vi "WM Dispersion Solver.vi"(1 "Gravity":dbl=9.806 min=1.0 format="%.3f", 2 "Water Depth":dbl=2.438 min=1e-16 format="%.3f", 3 "Wave Period":dbl=1.0 min=1e-16 format="%.3f") -> (0 "Wave Length":dbl format="%.3e")   [LabVIEW 2012]
uses:
  <vilib>/gmath/NI_Gmath.lvlib
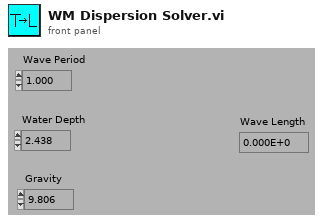
[diagram p1: front panel]
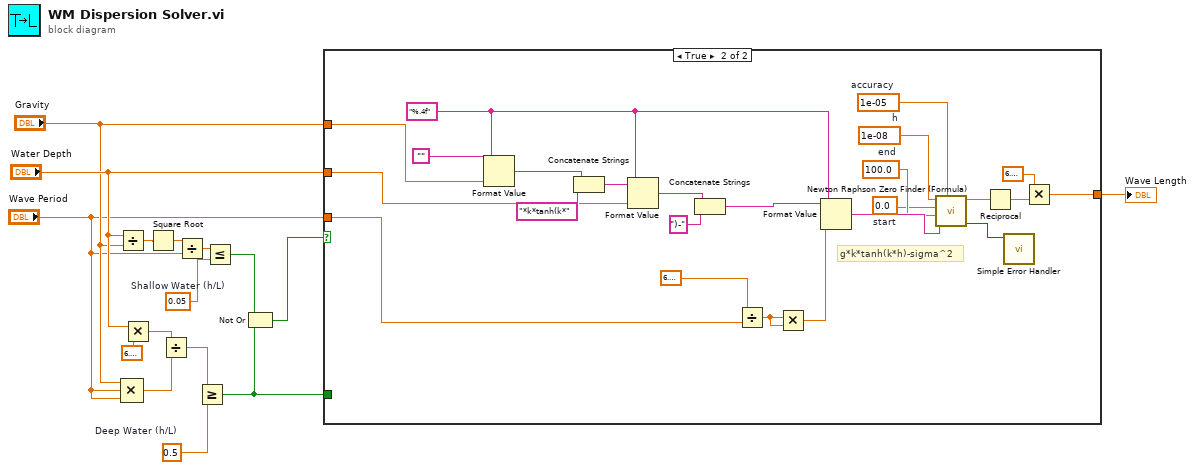
[diagram p0: block diagram]
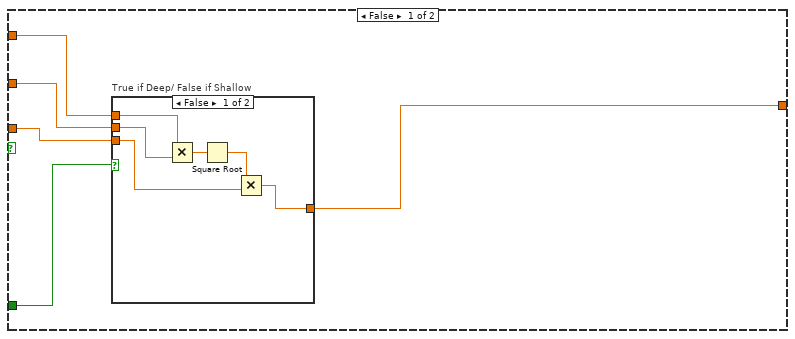
[diagram p2: hidden frame]
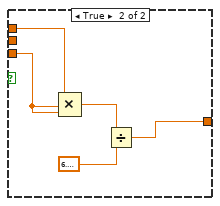
[diagram p3: hidden frame]
diagram:
  w5 = 0.5  # Deep Water (h/L)
  w12 = 0.05  # Shallow Water (h/L)
  n1 = Divide(x="Water Depth", y="Gravity") -> (x/y=w15:dbl)
  n2 = Compound Arithmetic op=MULTIPLY("Gravity", "Wave Period", "Wave Period") -> (w6:dbl)
  n3 = Multiply(x="Water Depth", y=6.283185307179586) -> (x*y=w9:dbl)
  n4 = Square Root(x=w15) -> (sqrt(x)=w14:dbl)
  n5 = Divide(x=w9, y=w6) -> (x/y=w4:dbl)
  n6 = Divide(x=w14, y="Wave Period") -> (x/y=w13:dbl)
  n7 = Greater Or Equal?(x=w4, y=w5) -> (x >= y?=w1:bool)
  n8 = Less Or Equal?(x=w13, y=w12) -> (x <= y?=w2:bool)
  n9 = Not Or(1:w1, 2:w2) -> (0:w3:bool)
  n10 = case shown="True" w3 {
    tunnel: "Wave Period" -> [w18 w55]
    tunnel: "Gravity" -> [w19 w51]
    tunnel: "Water Depth" -> [w17 w48]
    tunnel: [w20 w35] -> w16
    tunnel: w1 -> [w21 _]
    frame False {
      n11 = case "True if Deep/ False if Shallow" shown="False" w21 {
        tunnel: [w22 w28] -> w20
        tunnel: w19 -> [w27 w32]
        tunnel: w18 -> [w23 w31]
        tunnel: w17 -> [w26 _]
        frame False {
          n12 = Multiply(x=w27, y=w26) -> (x*y=w25:dbl)
          n13 = Square Root(x=w25) -> (sqrt(x)=w24:dbl)
          n14 = Multiply(x=w24, y=w23) -> (x*y=w22:dbl)
        }
        frame True {
          n15 = Compound Arithmetic op=MULTIPLY(w32, w31, w31) -> (w30:dbl)
          n16 = Divide(x=w30, y=6.283185307179586) -> (x/y=w28:dbl)
        }
      }
    }
    frame True {
      w33 = 1e-08  # h
      w34 = 1e-05  # accuracy
      w44 = "%.4f"
      w37 = 100.0  # end
      w36 = 0.0  # start
      # "g*k*tanh(k*h)-sigma^2"
      n17 = Format Value(string ("")="", format string=w44, value (0)=w51) -> (output string=w41:string)
      n18 = Concatenate Strings(w41, "*k*tanh(k*") -> (w49:string)
      n19 = Format Value(string ("")=w49, format string=w44, value (0)=w48) -> (output string=w47:string)
      n20 = Concatenate Strings(w47, ")-") -> (w45:string)
      n21 = Divide(x=6.283185307179586, y=w55) -> (x/y=w54:dbl)
      n22 = Multiply(x=w54, y=w54) -> (x*y=w52:dbl)
      n23 = Format Value(string ("")=w45, format string=w44, value (0)=w52) -> (output string=w38:string)
      n24 = call <vilib>:"Newton Raphson Zero Finder (Formula).vi"("accuracy"=w34, "formula"=w38, "end"=w37, "start"=w36, "h"=w33) -> ("error"=w53:i32, "zero"=w39:dbl)  [unwired: 3 in, 2 out]
      n25 = Reciprocal(x=w39) -> (1/x=w43:dbl)
      n26 = call <vilib>:"Simple Error Handler.vi"("error code (no error:0)"=w53) -> ()  [unwired: 4 in, 5 out]
      n27 = Multiply(x=6.283185307179586, y=w43) -> (x*y=w35:dbl)
    }
  }
  "Wave Length" <- w16
